vi "Get Reference.vi"(8 "Error In":errorcluster, 9 "Subpanel Ref":refnum<vi>, 11 "Test in":refnum<class "Test.lvclass">) -> (0 "Error Out":errorcluster, 3 "Test out":refnum<class "Test.lvclass">)   [LabVIEW 2020, in "Test.lvclass"]
doc: "Dynamic method to get the reference of asynchronously called VI for corresponding class"
uses:
  Test.lvclass
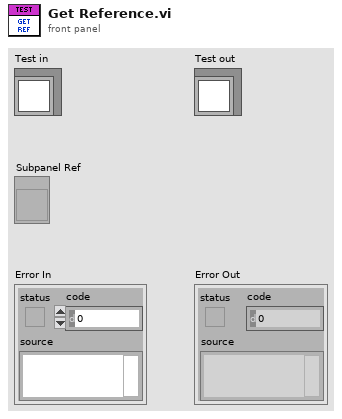
[diagram p1: front panel]
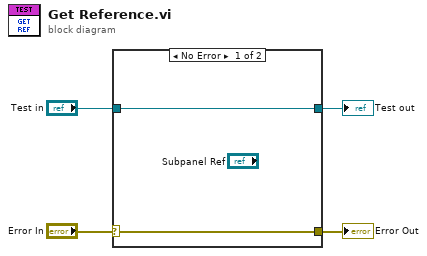
[diagram p0: block diagram]
diagram:
  n1 = case shown="No Error" "Error In" {
    selector: "Error In" -> [w5 w8]
    tunnel: [w5 w8] -> w3
    tunnel: [w6 w7] -> w1
    tunnel: "Test in" -> [w6 w7]
    frame No Error {
    }
    frame Error {
    }
  }
  "Error Out" <- w3
  "Test out" <- w1
